vi "Single_Core_Noise_Img_Gen-2.vi"(8 "error IN":errorcluster, 9 "[IN] Width":i32, 10 "[IN] Height":i32) -> (0 "error OUT":errorcluster, 2 "[OUT] U16 Pixel Img":u16[][](array[numeric]))   [LabVIEW 2020]
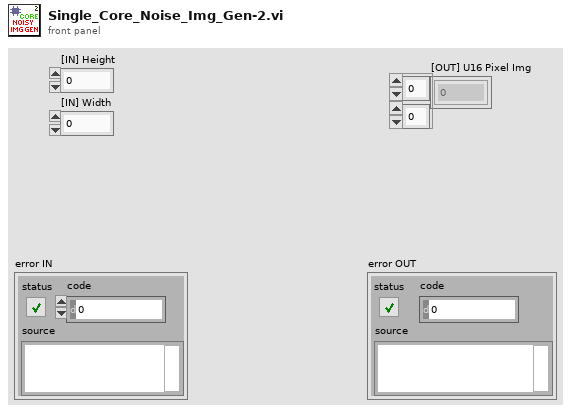
[diagram p1: front panel]
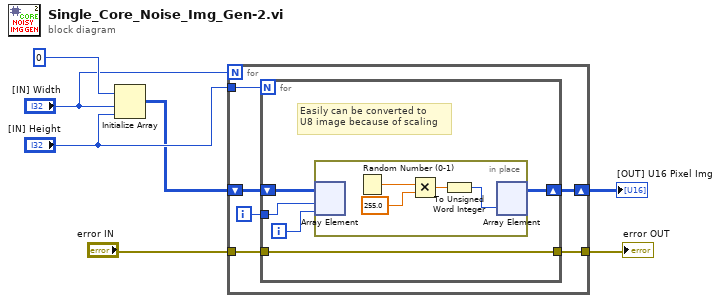
[diagram p0: block diagram]
diagram:
  n1 = Initialize Array(u16 0, "[IN] Width", "[IN] Height") -> (w4:u16[][])
  n2 = for {
    N: "[IN] Width" -> [_]
    tunnel: "error IN" -> [w13]
    tunnel: [w12] -> w1
    tunnel: "[IN] Height" -> [w11]
    shift-right: [w8] -> w2
    shift-left: w4 -> [w10]
    i -> [w9]
    n3 = for {
      N: w11 -> [_]
      tunnel: w13 -> [w18]
      tunnel: [w18] -> w12
      shift-right: [w14] -> w8
      shift-left: w10 -> [w17]
      tunnel: w9 -> [w15]
      i -> [w16]
      # "Easily can be converted to\nU8 image because of scaling"
      n4 = in-place {
        n5 = in-place-array #1(w17, w15, w16) -> ()  [unwired: 1 out]
        n6 = Random Number (0-1)() -> (number: 0 to 1=w20:dbl)
        n7 = Multiply(x=w20, y=255.0) -> (x*y=w21:dbl)
        n8 = To Unsigned Word Integer(number=w21) -> (unsigned 16bit integer=w19:u16)
        n9 = in-place-array #1(w19) -> (w14:u16[][])  [unwired: 2 out]
      }
    }
  }
  "error OUT" <- w1
  "[OUT] U16 Pixel Img" <- w2
